vi "CT-Initialize.vi"(0 "HCT Params":T1={"F0 (Hz)"=0.0, "Band"={"Flow (Hz)"=0.0, "Fhigh (Hz)"=0.0}, "Phase"=enum."Cosine", "Min F0 (Hz)"=0.0, "Max F0 (Hz)"=0.0, "ContinRandPhase"=FALSE, "Max peak factor"=inf, "Max mod depth"=2.0, "MinHarmNum"=0, "MaxHarmNum"=0, "Level Mode"=enum."per component", "% jitter"=0.0}, 7 "Fs (Hz)":dbl, 9 "Frame size (ms)":dbl, 11 "error in (no error)":errorcluster) -> (4 "CT Runtime":T3, 15 "error out":errorcluster)   [LabVIEW 2015]
uses:
  CT-Runtime Data.ctl
  CT-Params.ctl
  CT-Phase Enum.ctl
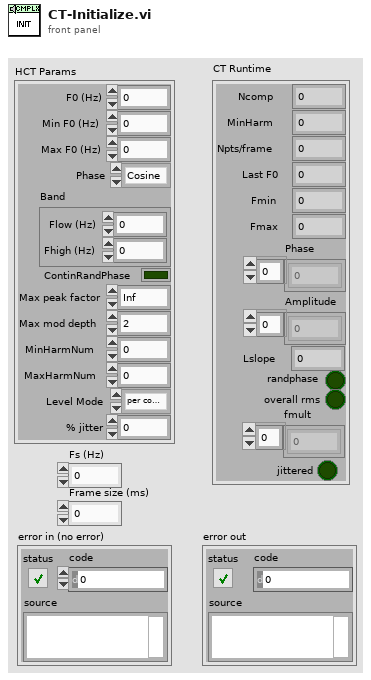
[diagram p1: front panel]
types:
  T1 = typedef "CT-Params.ctl" = cluster{"F0 (Hz)":dbl, "Band":cluster{"Flow (Hz)":dbl, "Fhigh (Hz)":dbl}, "Phase":T2, "Min F0 (Hz)":dbl, "Max F0 (Hz)":dbl, "ContinRandPhase":bool, "Max peak factor":dbl, "Max mod depth":dbl, "MinHarmNum":i32, "MaxHarmNum":i32, "Level Mode":enum16{"per component", "overall rms"}, "% jitter":dbl}
  T2 = typedef "CT-Phase Enum.ctl" = enum16{"Cosine", "Random", "Alternating"}
  T3 = typedef "CT-Runtime Data.ctl" = cluster{"Ncomp":i32, "MinHarm":i32, "Phase":dbl[], "Amplitude":dbl[], "Npts/frame":i32, "Last F0":dbl, "Fmin":dbl, "Fmax":dbl, "Lslope":dbl, "randphase":bool, "overall rms":bool, "fmult":dbl[], "jittered":bool}
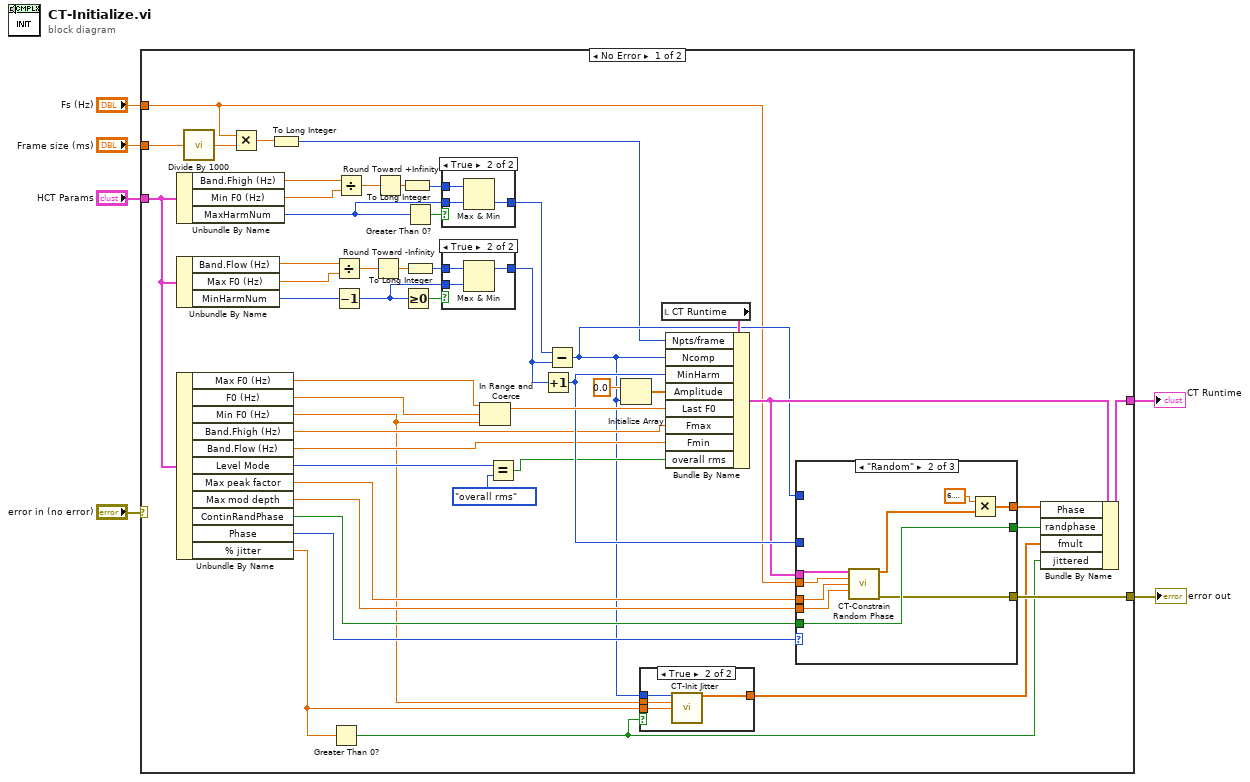
[diagram p0: block diagram]
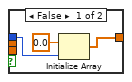
[diagram p2: hidden frame]
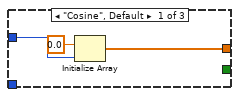
[diagram p5: hidden frame]
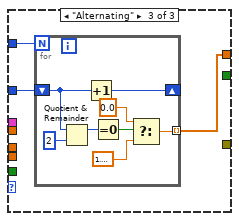
[diagram p6: hidden frame]
diagram:
  n1 = case shown="No Error" "error in (no error)" {
    selector: "error in (no error)" -> [_ w94]
    tunnel: "HCT Params" -> [w18 _]
    tunnel: [w44 _] -> w2
    tunnel: "Frame size (ms)" -> [w55 _]
    tunnel: "Fs (Hz)" -> [w10 _]
    tunnel: [w38 w94] -> w6
    frame No Error {
      n2 = Unbundle By Name(w18) -> ("Band.Fhigh (Hz)"=w35:dbl, "Min F0 (Hz)"=w34:dbl, "MaxHarmNum"=w31:i32)
      n3 = Unbundle By Name(w18) -> ("Band.Flow (Hz)"=w27:dbl, "Max F0 (Hz)"=w26:dbl, "MinHarmNum"=w23:i32)
      n4 = Unbundle By Name(w18) -> ("Max F0 (Hz)"=w48:dbl, "F0 (Hz)"=w49:dbl, "Min F0 (Hz)"=w9:dbl, "Band.Fhigh (Hz)"=w19:dbl, "Band.Flow (Hz)"=w20:dbl, "Level Mode"=w17:enum16{"per component", "overall rms"}, "Max peak factor"=w39:dbl, "Max mod depth"=w40:dbl, "ContinRandPhase"=w41:bool, "Phase"=w46:T2, "% jitter"=w8:dbl)
      n5 = call "Divide By 1000.vi"("X"=w55) -> ("X/1000"=w54:dbl)
      n6 = Multiply(x=w10, y=w54) -> (x*y=w51:dbl)
      n7 = To Long Integer(number=w51) -> (32bit integer=w12:i32)
      n8 = Greater Than 0?(x=w8) -> (x > 0?=w7:bool)
      n9 = Divide(x=w27, y=w26) -> (x/y=w29:dbl)
      n10 = Decrement(x=w23) -> (x-1=w22:i32)
      n11 = Divide(x=w35, y=w34) -> (x/y=w37:dbl)
      n12 = Round Toward -Infinity(1:w29) -> (0:w28:dbl)
      n13 = Round Toward +Infinity(x=w37) -> (ceil(x): smallest int >= x=w36:dbl)
      n14 = To Long Integer(number=w36) -> (32bit integer=w33:i32)
      n15 = Greater Or Equal To 0?(x=w22) -> (x >= 0?=w24:bool)
      n16 = Greater Than 0?(x=w31) -> (x > 0?=w32:bool)
      n17 = To Long Integer(number=w28) -> (32bit integer=w25:i32)
      n18 = case shown="True" w32 {
        tunnel: w33 -> [w67 w70]
        tunnel: w31 -> [_ w69]
        tunnel: [w67 w68] -> w30
        frame False {
        }
        frame True {
          n19 = Max & Min(x=w70, y=w69) -> (min(x,y)=w68:i32)  [unwired: 1 out]
        }
      }
      n20 = case shown="True" w24 {
        tunnel: w25 -> [w63 w66]
        tunnel: w22 -> [_ w65]
        tunnel: [w63 w64] -> w21
        frame False {
        }
        frame True {
          n21 = Max & Min(x=w66, y=w65) -> (max(x,y)=w64:i32)  [unwired: 1 out]
        }
      }
      n22 = In Range and Coerce(upper limit=w48, x=w49, lower limit=w9) -> (coerced(x)=w50:dbl)  [unwired: 1 out]
      n23 = Equal?(x=w17, y=enum16{"per component", "overall rms"}."overall rms") -> (x = y?=w15:bool)
      n24 = Increment(x=w21) -> (x+1=w45:i32)
      n25 = Subtract(x=w30, y=w21) -> (x-y=w14:i32)
      n26 = Initialize Array(0.0 ("element"), w14) -> (w52:dbl[])
      n27 = case shown="True" w7 {
        tunnel: w14 -> [w57 w62]
        tunnel: [w58 w61] -> w13
        tunnel: w9 -> [_ w60]
        tunnel: w8 -> [_ w59]
        frame False {
          n28 = Initialize Array(0.0 ("element"), w57) -> (w58:dbl[])
        }
        frame True {
          n29 = call "CT-Init Jitter.vi"("Num Components"=w62, "Min F0 (Hz)"=w60, "% jitter"=w59) -> ("frequency multipliers"=w61:dbl[])  [unwired: 12 in]
        }
      }
      n30 = local read "CT Runtime"() -> (w47:T3)
      n31 = Bundle By Name(cluster=w47, "Npts/frame"=w12, "Ncomp"=w14, "MinHarm"=w45, "Amplitude"=w52, "Last F0"=w50, "Fmax"=w19, "Fmin"=w20, "overall rms"=w15) -> (w42:T3)
      n32 = case shown="\"Random\"" w46 {
        tunnel: w14 -> [w72 _ w85]
        tunnel: w45 -> [_ _ w84]
        tunnel: [w71 w81 w83] -> w11
        tunnel: [_ w80 _] -> w43
        tunnel: w41 -> [_ w80 _]
        tunnel: w42 -> [_ w79 _]
        tunnel: w10 -> [_ w78 _]
        tunnel: w40 -> [_ w75 _]
        tunnel: w39 -> [_ w76 _]
        tunnel: [_ w74 _] -> w38
        frame "Cosine", Default {
          n33 = Initialize Array(0.0 ("element"), w72) -> (w71:dbl[])
        }
        frame "Random" {
          n34 = call "CT-Constrain Random Phase.vi"("HCT Runtime"=w79, "Fs (Hz)"=w78, "Max peak factor"=w76, "Max mod depth"=w75) -> ("Phase"=w77:dbl[], "error out"=w74:errorcluster)  [unwired: 10 in]
          n35 = Multiply(x=6.283185307179586, y=w77) -> (x*y=w81:dbl[])
        }
        frame "Alternating" {
          n36 = for {
            N: w85 -> [_]
            shift-right: [w93] -> _
            shift-left: w84 -> [w92]
            tunnel: [w86] -> w83 mode=indexing
            n37 = Quotient & Remainder(x=w92, y=2) -> (x-y*floor(x/y)=w90:i32)  [unwired: 1 out]
            n38 = Increment(x=w92) -> (x+1=w93:i32)
            n39 = Equal To 0?(x=w90) -> (x = 0?=w89:bool)
            n40 = Select(t=0.0, s=w89, f=1.5707963267948966) -> (s? t:f=w86:dbl)
          }
        }
      }
      n41 = Bundle By Name(cluster=w42, "Phase"=w11, "randphase"=w43, "fmult"=w13, "jittered"=w7) -> (w44:T3)
    }
    frame Error {
    }
  }
  "error out" <- w6
  "CT Runtime" <- w2
